vi "申请通道.vi"(9 "通道":string, 11 "TCP Network Connection in":refnum<k5>) -> (0 "error out":errorcluster, 1 "ack":string, 3 "TCP Network Connection out":refnum<k5>)   [LabVIEW 2015]
uses:
  Global/SeverGlobal.vi
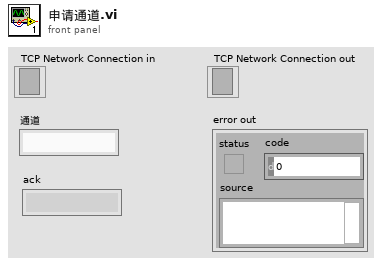
[diagram p1: front panel]
types:
  T1 = typedef "响应消息头.ctl" = string
  T2 = cluster{"TCP Ref":refnum<k5>, "IP":string, "userName":string, "A":u16, "COM":u16, "time":u32}[]
  T3 = cluster{"TCP Ref":refnum<k5>, "Broadcast":refnum<k5>, "TF Ref":refnum<k5>, "IP":string, "port":u16, "userName":string, "passWord":string, "authority":string}[]
  T4 = cluster{"TCP Ref":refnum<k5>, "IP":string, "userName":string, "A":u16, "COM":u16, "time":u32}
  T5 = typedef "队列.ctl" = cluster{"COM1":refnum<queue>, "COM2":refnum<queue>, "COM3":refnum<queue>, "COM4":refnum<queue>, "OUT1":refnum<queue>, "OUT2":refnum<queue>, "OUT3":refnum<queue>, "OUT4":refnum<queue>, "OUT5":refnum<queue>, "OUT6":refnum<queue>, "OUT7":refnum<queue>, "OUT8":refnum<queue>}
  T6 = cluster{"TCP Ref":refnum<k5>, "IP":string, "userName":string, "IN":u16, "OUT":u16, "time":u32}[]
  T7 = cluster{"TCP Ref":refnum<k5>, "IP":string, "userName":string, "IN":u16, "OUT":u16, "time":u32}
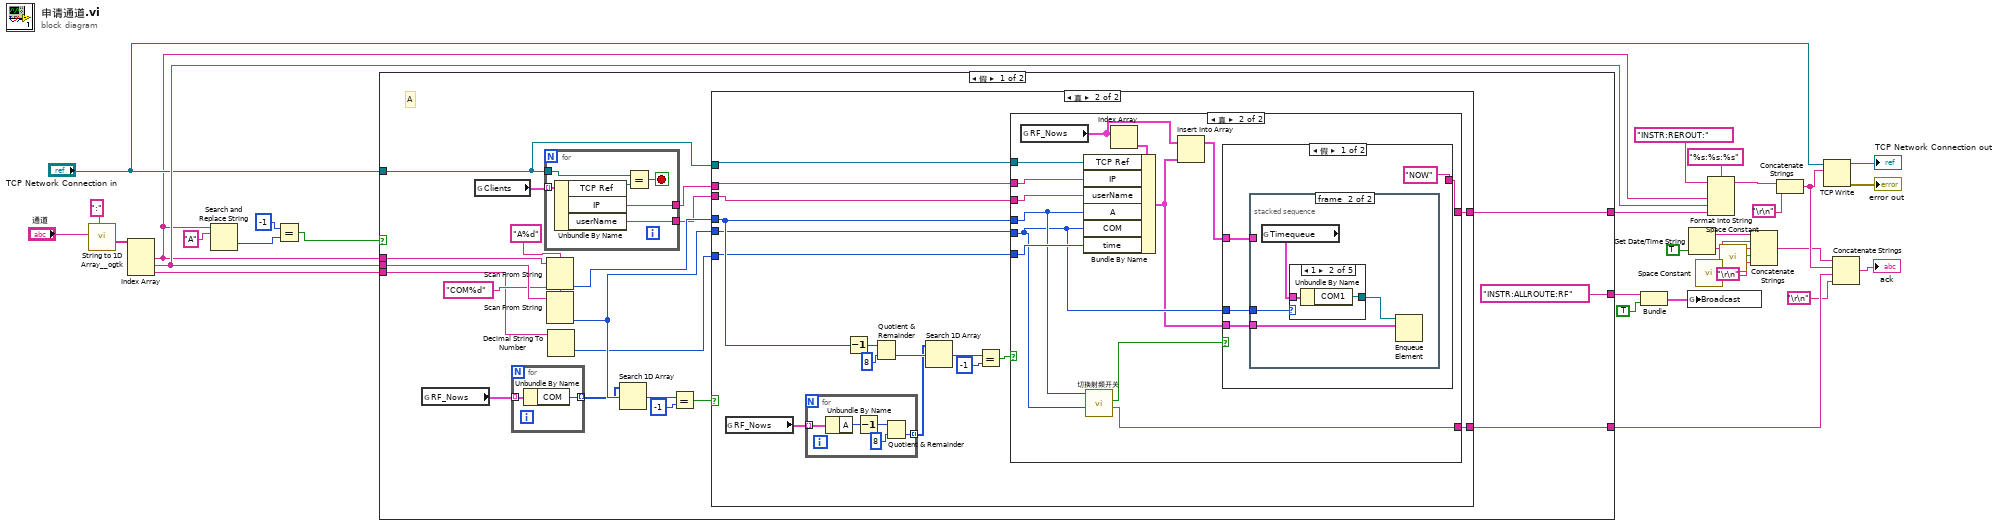
[diagram p0: block diagram]
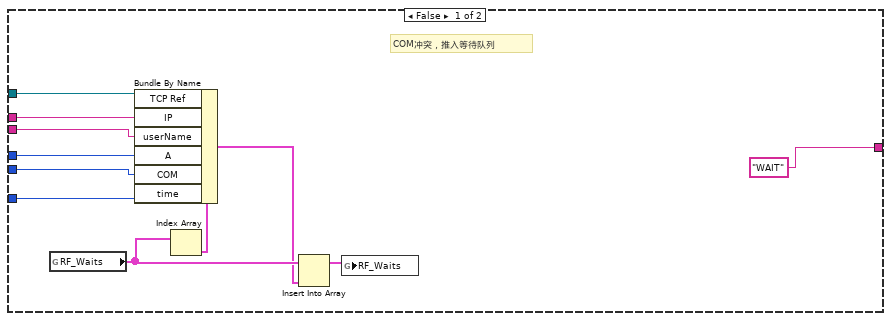
[diagram p2: hidden frame]
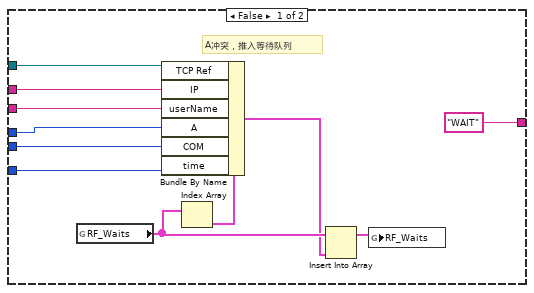
[diagram p3: hidden frame]
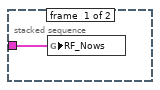
[diagram p4: hidden frame]
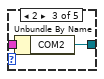
[diagram p6: hidden frame]
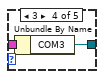
[diagram p7: hidden frame]
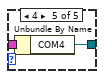
[diagram p8: hidden frame]
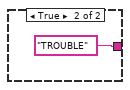
[diagram p9: hidden frame]
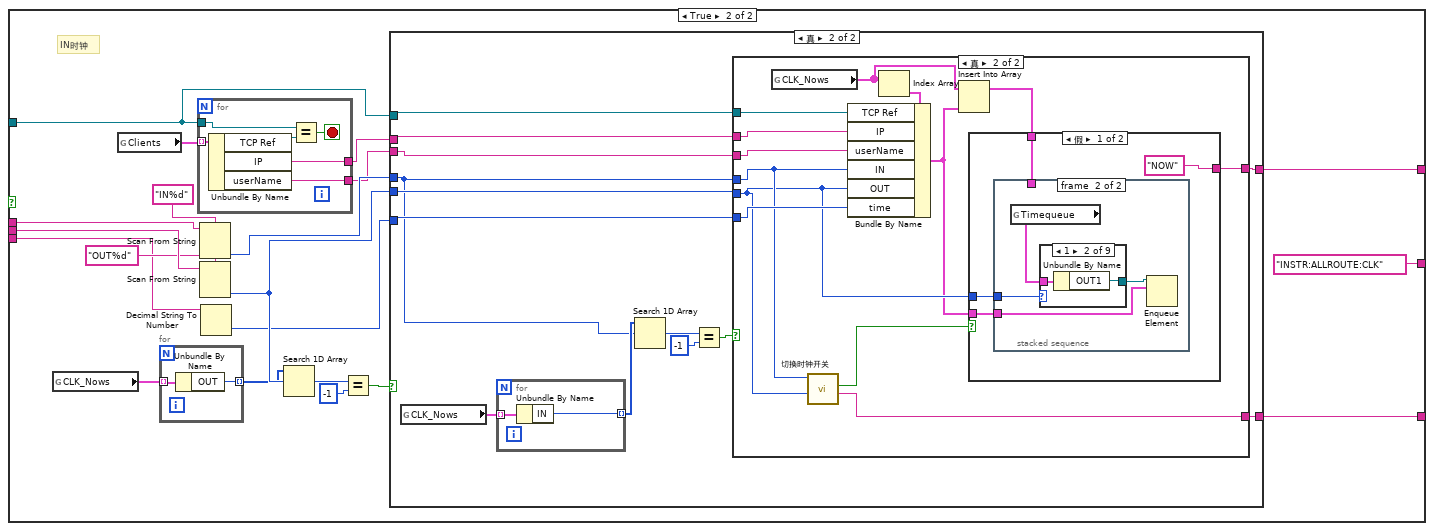
[diagram p10: hidden frame]
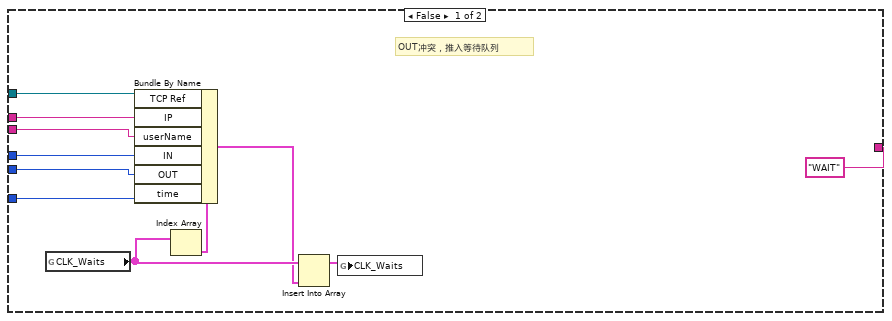
[diagram p11: hidden frame]
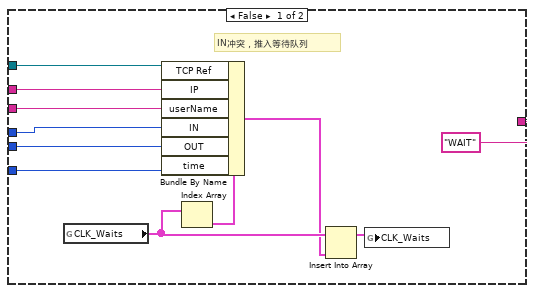
[diagram p12: hidden frame]
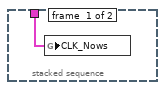
[diagram p13: hidden frame]
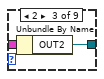
[diagram p15: hidden frame]
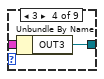
[diagram p16: hidden frame]
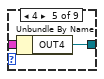
[diagram p17: hidden frame]
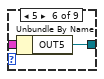
[diagram p18: hidden frame]
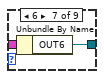
[diagram p19: hidden frame]
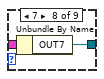
[diagram p20: hidden frame]
diagram:
  n1 = call <userlib>:"String to 1D Array__ogtk.vi"("delimiter (Tab)"=":", "string"="通道") -> ("Array of Strings"=w22:string[])  [unwired: 9 in]
  n2 = Index Array(array=w22) -> (element #1=w19:string, element #2=w32:string, element #3=w24:string)  [unwired: 3 in]
  n3 = Search and Replace String(input string=w19, search string="A") -> (offset past replacement=w17:i32)  [unwired: 6 in, 3 out]
  n4 = Equal?(x=-1, y=w17) -> (x = y?=w15:bool)
  n5 = case shown="假" w15 {
    tunnel: w32 -> [w52 w154]
    tunnel: w19 -> [w51 w153]
    tunnel: [w46 w148] -> w31
    tunnel: w24 -> [w44 w146]
    tunnel: "TCP Network Connection in" -> [w35 w137]
    tunnel: ["INSTR:ALLROUTE:RF" "INSTR:ALLROUTE:CLK"] -> w12
    tunnel: [w33 w135] -> w9
    frame False {
      # "A"
      n6 = global read "SeverGlobal.vi" "RF_Nows"() -> (w36:T2)
      n7 = global read "SeverGlobal.vi" "Clients"() -> (w41:T3)
      n8 = for {
        tunnel: w36 -> [w134] mode=indexing
        tunnel: [w133] -> w37 mode=indexing
        n9 = Unbundle By Name(w134) -> ("COM"=w133:u16)
      }
      n10 = for {
        tunnel: w41 -> [w58] mode=indexing
        tunnel: w35 -> [w56]
        tunnel: [w54] -> w42
        tunnel: [w53] -> w43
        stop <- w55 stop-if-true
        n11 = Unbundle By Name(w58) -> ("TCP Ref"=w57:refnum<k5>, "IP"=w54:string, "userName"=w53:string)
        n12 = Equal?(x=w56, y=w57) -> (x = y?=w55:bool)
      }
      n13 = Scan From String(format string="A%d", input string=w51) -> (output 1=w47:i32)  [unwired: 3 in, 3 out]
      n14 = Scan From String(format string="COM%d", input string=w52) -> (output 1=w49:i32)  [unwired: 3 in, 3 out]
      n15 = Decimal String To Number(string=w44) -> (number=w45:i32)  [unwired: 2 in, 1 out]
      n16 = Search 1D Array(1D array=w37, element=w49) -> (index of element=w39:i32)  [unwired: 1 in]
      n17 = Equal?(x=w39, y=-1) -> (x = y?=w40:bool)
      n18 = case shown="真" w40 {
        tunnel: w35 -> [w65 w79]
        tunnel: w42 -> [w64 w78]
        tunnel: w43 -> [w63 w77]
        tunnel: w47 -> [w62 w76]
        tunnel: w49 -> [w61 w75]
        tunnel: w45 -> [w60 w74]
        tunnel: ["WAIT" w71] -> w46
        tunnel: [_ w70] -> w33
        frame False {
          # "COM冲突，推入等待队列"
          n19 = global read "SeverGlobal.vi" "RF_Waits"() -> (w68:T2)
          n20 = Index Array(array=w68) -> (element=w67:T4)  [unwired: 1 in]
          n21 = Bundle By Name(cluster=w67, "TCP Ref"=w65, "IP"=w64, "userName"=w63, "A"=w62, "COM"=w61, "time"=w60) -> (w66:T4)
          n22 = Insert Into Array(array=w68, new element=w66) -> (w69:T2)  [unwired: 1 in]
          n23 = global write "SeverGlobal.vi" "RF_Waits"(w69) -> ()
        }
        frame True {
          n24 = global read "SeverGlobal.vi" "RF_Nows"() -> (w73:T2)
          n25 = for {
            tunnel: w73 -> [w90] mode=indexing
            tunnel: [w86] -> w72 mode=indexing
            n26 = Unbundle By Name(w90) -> ("A"=w87:u16)
            n27 = Decrement(x=w87) -> (x-1=w88:u16)
            n28 = Quotient & Remainder(x=w88, y=8) -> (floor(x/y)=w86:i32)  [unwired: 1 out]
          }
          n29 = Decrement(x=w76) -> (x-1=w85:i32)
          n30 = Quotient & Remainder(x=w85, y=8) -> (floor(x/y)=w81:i32)  [unwired: 1 out]
          n31 = Search 1D Array(1D array=w72, element=w81) -> (index of element=w83:i32)  [unwired: 1 in]
          n32 = Equal?(x=w83, y=-1) -> (x = y?=w80:bool)
          n33 = case shown="真" w80 {
            tunnel: w79 -> [w97 w108]
            tunnel: w78 -> [w96 w112]
            tunnel: w77 -> [w95 w111]
            tunnel: w76 -> [w94 w107]
            tunnel: w75 -> [w93 w103]
            tunnel: w74 -> [w92 w110]
            tunnel: ["WAIT" w109] -> w71
            tunnel: [_ w106] -> w70
            frame False {
              # "A冲突，推入等待队列"
              n34 = global read "SeverGlobal.vi" "RF_Waits"() -> (w100:T2)
              n35 = Index Array(array=w100) -> (element=w99:T4)  [unwired: 1 in]
              n36 = Bundle By Name(cluster=w99, "TCP Ref"=w97, "IP"=w96, "userName"=w95, "A"=w94, "COM"=w93, "time"=w92) -> (w98:T4)
              n37 = Insert Into Array(array=w100, new element=w98) -> (w101:T2)  [unwired: 1 in]
              n38 = global write "SeverGlobal.vi" "RF_Waits"(w101) -> ()
            }
            frame True {
              n39 = global read "SeverGlobal.vi" "RF_Nows"() -> (w114:T2)
              n40 = call "切换射频开关.vi"("COM"=w103, "A"=w107) -> ("ask"=w106:string, "Isfailed"=w105:bool)  [unwired: 7 in, 1 out]
              n41 = Index Array(array=w114) -> (element=w113:T4)  [unwired: 1 in]
              n42 = Bundle By Name(cluster=w113, "TCP Ref"=w108, "IP"=w112, "userName"=w111, "A"=w107, "COM"=w103, "time"=w110) -> (w102:T4)
              n43 = Insert Into Array(array=w114, new element=w102) -> (w104:T2)  [unwired: 1 in]
              n44 = case shown="假" w105 {
                tunnel: ["NOW" "TROUBLE"] -> w109
                tunnel: w104 -> [w117 _]
                tunnel: w103 -> [w116 _]
                tunnel: w102 -> [w115 _]
                frame False {
                  n45 = stacked-sequence {
                    tunnel: w117 -> [w119 _]
                    tunnel: w116 -> [_ w121]
                    tunnel: w115 -> [_ w120]
                    frame #0 {
                      n46 = global write "SeverGlobal.vi" "RF_Nows"(w119) -> ()
                    }
                    frame #1 {
                      n47 = global read "SeverGlobal.vi" "Timequeue"() -> (w123:T5)
                      n48 = case shown="1" w121 {
                        tunnel: w123 -> [_ w125 w127 w129 w131]
                        tunnel: [_ w124 w126 w128 w130] -> w122
                        frame 0, Default {
                        }
                        frame 1 {
                          n49 = Unbundle By Name(w125) -> ("COM1"=w124:refnum<queue>)
                        }
                        frame 2 {
                          n50 = Unbundle By Name(w127) -> ("COM2"=w126:refnum<queue>)
                        }
                        frame 3 {
                          n51 = Unbundle By Name(w129) -> ("COM3"=w128:refnum<queue>)
                        }
                        frame 4 {
                          n52 = Unbundle By Name(w131) -> ("COM4"=w130:refnum<queue>)
                        }
                      }
                      n53 = Enqueue Element(queue=w122, element=w120) -> ()  [unwired: 2 in, 3 out]
                    }
                  }
                }
                frame True {
                }
              }
            }
          }
        }
      }
    }
    frame True {
      # "IN时钟"
      n54 = global read "SeverGlobal.vi" "CLK_Nows"() -> (w138:T6)
      n55 = global read "SeverGlobal.vi" "Clients"() -> (w143:T3)
      n56 = for {
        tunnel: w138 -> [w238] mode=indexing
        tunnel: [w237] -> w139 mode=indexing
        n57 = Unbundle By Name(w238) -> ("OUT"=w237:u16)
      }
      n58 = for {
        tunnel: w143 -> [w160] mode=indexing
        tunnel: w137 -> [w158]
        tunnel: [w156] -> w144
        tunnel: [w155] -> w145
        stop <- w157 stop-if-true
        n59 = Unbundle By Name(w160) -> ("TCP Ref"=w159:refnum<k5>, "IP"=w156:string, "userName"=w155:string)
        n60 = Equal?(x=w158, y=w159) -> (x = y?=w157:bool)
      }
      n61 = Scan From String(format string="IN%d", input string=w153) -> (output 1=w149:i32)  [unwired: 3 in, 3 out]
      n62 = Scan From String(format string="OUT%d", input string=w154) -> (output 1=w151:i32)  [unwired: 3 in, 3 out]
      n63 = Decimal String To Number(string=w146) -> (number=w147:i32)  [unwired: 2 in, 1 out]
      n64 = Search 1D Array(1D array=w139, element=w151) -> (index of element=w141:i32)  [unwired: 1 in]
      n65 = Equal?(x=w141, y=-1) -> (x = y?=w142:bool)
      n66 = case shown="真" w142 {
        tunnel: w137 -> [w167 w181]
        tunnel: w144 -> [w166 w180]
        tunnel: w145 -> [w165 w179]
        tunnel: w149 -> [w164 w173]
        tunnel: w151 -> [w163 w178]
        tunnel: w147 -> [w162 w177]
        tunnel: ["WAIT" w174] -> w148
        tunnel: [_ w172] -> w135
        frame False {
          # "OUT冲突，推入等待队列"
          n67 = global read "SeverGlobal.vi" "CLK_Waits"() -> (w170:T6)
          n68 = Index Array(array=w170) -> (element=w169:T7)  [unwired: 1 in]
          n69 = Bundle By Name(cluster=w169, "TCP Ref"=w167, "IP"=w166, "userName"=w165, "IN"=w164, "OUT"=w163, "time"=w162) -> (w168:T7)
          n70 = Insert Into Array(array=w170, new element=w168) -> (w171:T6)  [unwired: 1 in]
          n71 = global write "SeverGlobal.vi" "CLK_Waits"(w171) -> ()
        }
        frame True {
          n72 = global read "SeverGlobal.vi" "CLK_Nows"() -> (w176:T6)
          n73 = for {
            tunnel: w176 -> [w186] mode=indexing
            tunnel: [w185] -> w175 mode=indexing
            n74 = Unbundle By Name(w186) -> ("IN"=w185:u16)
          }
          n75 = Search 1D Array(1D array=w175, element=w173) -> (index of element=w184:i32)  [unwired: 1 in]
          n76 = Equal?(x=w184, y=-1) -> (x = y?=w182:bool)
          n77 = case shown="真" w182 {
            tunnel: w181 -> [w193 w205]
            tunnel: w180 -> [w192 w208]
            tunnel: w179 -> [w191 w207]
            tunnel: w173 -> [w190 w204]
            tunnel: w178 -> [w189 w199]
            tunnel: w177 -> [w188 w206]
            tunnel: ["WAIT" w203] -> w174
            tunnel: [_ w202] -> w172
            frame False {
              # "IN冲突，推入等待队列"
              n78 = global read "SeverGlobal.vi" "CLK_Waits"() -> (w196:T6)
              n79 = Index Array(array=w196) -> (element=w195:T7)  [unwired: 1 in]
              n80 = Bundle By Name(cluster=w195, "TCP Ref"=w193, "IP"=w192, "userName"=w191, "IN"=w190, "OUT"=w189, "time"=w188) -> (w194:T7)
              n81 = Insert Into Array(array=w196, new element=w194) -> (w197:T6)  [unwired: 1 in]
              n82 = global write "SeverGlobal.vi" "CLK_Waits"(w197) -> ()
            }
            frame True {
              n83 = global read "SeverGlobal.vi" "CLK_Nows"() -> (w210:T6)
              n84 = call "切换时钟开关.vi"("OUT"=w199, "IN"=w204) -> ("ask"=w202:string, "Isfailed"=w201:bool)  [unwired: 7 in, 1 out]
              n85 = Index Array(array=w210) -> (element=w209:T7)  [unwired: 1 in]
              n86 = Bundle By Name(cluster=w209, "TCP Ref"=w205, "IP"=w208, "userName"=w207, "IN"=w204, "OUT"=w199, "time"=w206) -> (w198:T7)
              n87 = Insert Into Array(array=w210, new element=w198) -> (w200:T6)  [unwired: 1 in]
              n88 = case shown="假" w201 {
                tunnel: ["NOW" "TROUBLE"] -> w203
                tunnel: w200 -> [w213 _]
                tunnel: w199 -> [w212 _]
                tunnel: w198 -> [w211 _]
                frame False {
                  n89 = stacked-sequence {
                    tunnel: w212 -> [_ w217]
                    tunnel: w211 -> [_ w216]
                    tunnel: w213 -> [w215 _]
                    frame #0 {
                      n90 = global write "SeverGlobal.vi" "CLK_Nows"(w215) -> ()
                    }
                    frame #1 {
                      n91 = global read "SeverGlobal.vi" "Timequeue"() -> (w219:T5)
                      n92 = case shown="1" w217 {
                        tunnel: w219 -> [_ w221 w223 w225 w227 w229 w231 w233 w235]
                        tunnel: [_ w220 w222 w224 w226 w228 w230 w232 w234] -> w218
                        frame 0, Default {
                        }
                        frame 1 {
                          n93 = Unbundle By Name(w221) -> ("OUT1"=w220:refnum<queue>)
                        }
                        frame 2 {
                          n94 = Unbundle By Name(w223) -> ("OUT2"=w222:refnum<queue>)
                        }
                        frame 3 {
                          n95 = Unbundle By Name(w225) -> ("OUT3"=w224:refnum<queue>)
                        }
                        frame 4 {
                          n96 = Unbundle By Name(w227) -> ("OUT4"=w226:refnum<queue>)
                        }
                        frame 5 {
                          n97 = Unbundle By Name(w229) -> ("OUT5"=w228:refnum<queue>)
                        }
                        frame 6 {
                          n98 = Unbundle By Name(w231) -> ("OUT6"=w230:refnum<queue>)
                        }
                        frame 7 {
                          n99 = Unbundle By Name(w233) -> ("OUT7"=w232:refnum<queue>)
                        }
                        frame 8 {
                          n100 = Unbundle By Name(w235) -> ("OUT8"=w234:refnum<queue>)
                        }
                      }
                      n101 = Enqueue Element(queue=w218, element=w216) -> ()  [unwired: 2 in, 3 out]
                    }
                  }
                }
                frame True {
                }
              }
            }
          }
        }
      }
    }
  }
  n102 = Bundle(w12, TRUE) -> (w14:cluster{string, bool})  [unwired: 1 in]
  n103 = global write "SeverGlobal.vi" "Broadcast"(w14) -> ()
  n104 = Get Date/Time String(want seconds? (F)=TRUE ("需要秒？(F)")) -> (date string=w7:string, time string=w6:string)  [unwired: 2 in]
  n105 = call <vilib>:"Space Constant.vi"() -> ("String"=w5:string)
  n106 = Format Into String(format string="%s:%s:%s", initial string=T1 "INSTR:REROUT:" ("Combo Box"), w19, w32, w31) -> (resulting string=w30:string)  [unwired: 1 in, 1 out]
  n107 = call <vilib>:"Space Constant.vi"() -> ("String"=w4:string)
  n108 = Concatenate Strings(w7, w5, w6, w4, "\r\n") -> (w2:string)
  n109 = Concatenate Strings(w30, "\r\n") -> (w10:string)
  n110 = TCP Write(connection ID="TCP Network Connection in", data in=w10) -> (connection ID out=→"TCP Network Connection out":refnum<k5>, error out=→"error out":errorcluster)  [unwired: 2 in, 1 out]
  n111 = Concatenate Strings(w2, w10, w9, "\r\n") -> (→"ack":string)
